vi "Find Flags.vi"(8 "error in":errorcluster, 11 "Image In":T1) -> (0 "error out":errorcluster, 1 "Blue Flag":cluster{"X Centroid":sgl, "Y Centroid":sgl} {"Y Centroid" format="%.2f"; "X Centroid" format="%.2f"}, 2 "Red Flag":cluster{"X Centroid":sgl, "Y Centroid":sgl} {"Y Centroid" format="%.2f"; "X Centroid" format="%.2f"}, 3 "Image Out":T1)   [LabVIEW 2012]
uses:
  <vilib>/vision/Image Controls.llb/IMAQ Image.ctl
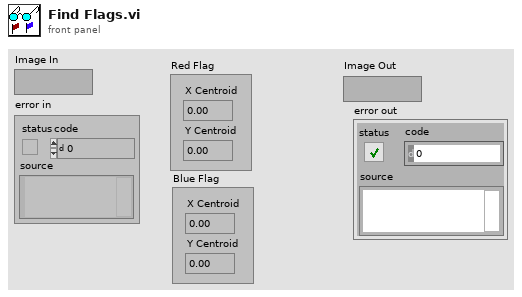
[diagram p1: front panel]
types:
  T1 = typedef "IMAQ Image.ctl" = refnum<image>
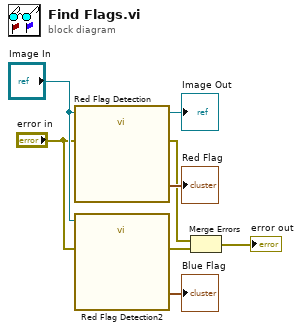
[diagram p0: block diagram]
diagram:
  n1 = call "Red Flag Detection"("Image In"="Image In", "error in"="error in") -> ("Image Out"=→"Image Out":T1, "Calibrated Centroid (Centroid 1)"=→"Red Flag":cluster{"X Centroid":sgl, "Y Centroid":sgl}, "error out"=w4:errorcluster)  [unwired: 23 in]
  n2 = call "Red Flag Detection2"("Image In"="Image In", "error in"="error in") -> ("Calibrated Centroid (Centroid 1)"=→"Blue Flag":cluster{"X Centroid":sgl, "Y Centroid":sgl}, "error out"=w3:errorcluster)  [unwired: 23 in, 1 out]
  n3 = Merge Errors(w4, w3) -> (→"error out":errorcluster)
